vi "Host_HealthCheck_update.vi"(0 "reference in":refnum<vi>, 1 "input cluster":T1={"cRIO Data"={"Time (ms)"=0.0, "24V Battery (V)"=0.0, "LowV Current (A)"=0.0, "Fiducial Sensor (V)"=0.0, "PV Pressure (psig)"=0.0, "Flow Sensor (V)"=0.0, "Temp Fairing (F)"=0.0, "Temp Reservoir (F)"=0.0, "HallEffect Right (in)"=0.0, "HallEffect Left (in)"=0.0, "PT Tank (psig)"=0.0, "PT Clamp Right (psig)"=0.0, "PT Clamp Left (psig)"=0.0, "PT Brake (psig)"=0.0, "PT Cooling (psig)"=0.0, "Displacement (ft)"=0.0, "Velocity (ft/s)"=0.0}, "IMU Data"={"x acceleration (g)"=0.0, "Pressure (psia)"=0.0, "Temperature (F)"=0.0}, "BMS Data"={"Max Cell Voltage (V)"=0.0, "Max Cell ID"=0.0, "Min Cell Voltage (V)"=0.0, "Min Cell ID"=0.0, "State of Charge (%)"=0.0, "Average Voltage (V)"=0.0, "Voltage Delta (V)"=0.0, "Pack Current (A)"=0.0, "Pack Voltage (V)"=0.0, "Max Resistance (Ohm)"=0.0, "Min Resistance (Ohm)"=0.0, "Average Resistance (Ohm)"=0.0, "Delta Resistance (Ohm)"=0.0, "Highest Temperature(F)"=0.0, "BmsStatus"={"isFault"=FALSE, "isolationMonitoring"=FALSE}}, "Motor Data"={"Velo (RPM)"=0.0, "MotorTemp(F)"=0.0, "CtrlTemp(F)"=0.0, "DcLinkVolt(V)"=0.0, "ErrorCode"=0.0, "motorStatus"={"isReady"=FALSE, "isOn"=FALSE, "isOperEn"=FALSE, "isFault"=FALSE, "isVoltEn"=FALSE, "targetReached"=FALSE, "isWarning"=FALSE}, "isAlive"=FALSE, "motorControllerState"=1}} {"Motor Data"."motorControllerState" items=["unknown"=1, "boot-up"=0, "stopped"=4, "operational"=5, "pre-operational"=127, "connection lost"=128]}) -> ()   [LabVIEW 2017]
doc: "Updates Health Check Display\nIN: Table, Sensor Data\nOUT: Updated Table"
uses:
  Master/DAQ/Master_DataControl.ctl
  Master/DAQ/TypeDef_cRIOData.ctl
  Master/IMU/TypeDef_IMUData.ctl
  Master/CAN/TypeDef_BMSData.ctl
  Master/CAN/TypeDef_BMS_Status.ctl
  Master/CAN/MotorController/fixedMotorData.ctl
  Master/CAN/MotorController/MotorStatus.ctl
  <vilib>/Utility/miscctls.llb/LVRowAndColumnTypeDef.ctl
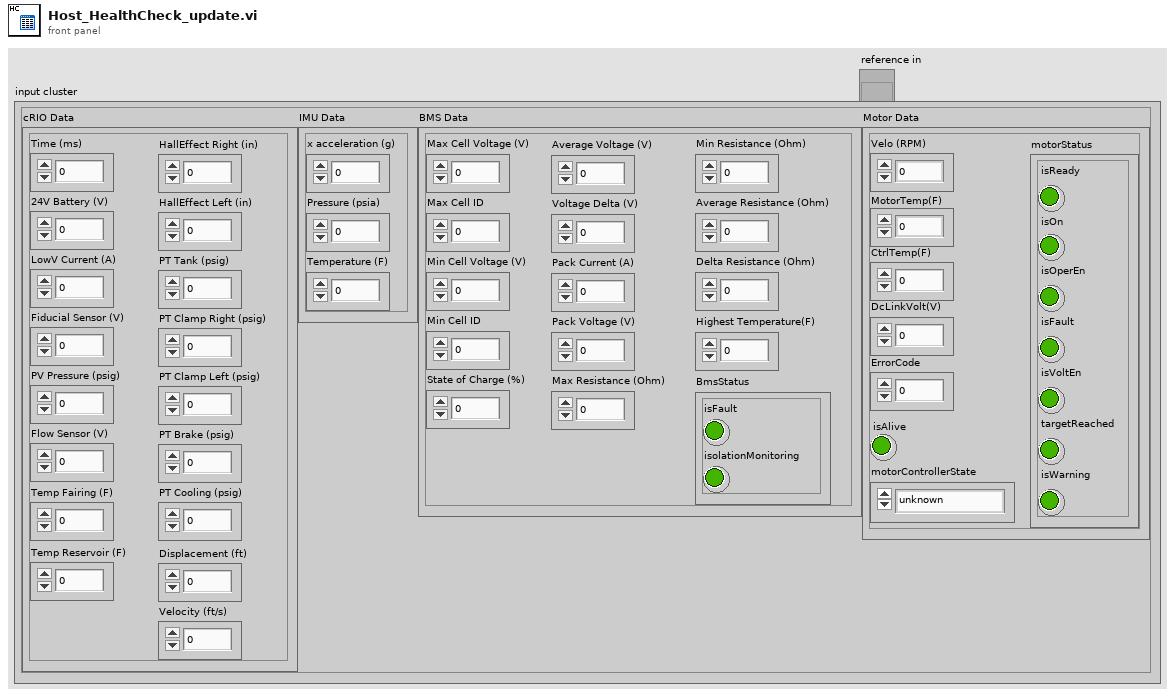
[diagram p1: front panel]
types:
  T1 = typedef "Master_DataControl.ctl" = cluster{"cRIO Data":T2, "IMU Data":T3, "BMS Data":T4, "Motor Data":T6}
  T2 = typedef "TypeDef_cRIOData.ctl" = cluster{"Time (ms)":dbl, "24V Battery (V)":dbl, "LowV Current (A)":dbl, "Fiducial Sensor (V)":dbl, "PV Pressure (psig)":dbl, "Flow Sensor (V)":dbl, "Temp Fairing (F)":dbl, "Temp Reservoir (F)":dbl, "HallEffect Right (in)":dbl, "HallEffect Left (in)":dbl, "PT Tank (psig)":dbl, "PT Clamp Right (psig)":dbl, "PT Clamp Left (psig)":dbl, "PT Brake (psig)":dbl, "PT Cooling (psig)":dbl, "Displacement (ft)":dbl, "Velocity (ft/s)":dbl}
  T3 = typedef "TypeDef_IMUData.ctl" = cluster{"x acceleration (g)":dbl, "Pressure (psia)":dbl, "Temperature (F)":dbl}
  T4 = typedef "TypeDef_BMSData.ctl" = cluster{"Max Cell Voltage (V)":dbl, "Max Cell ID":dbl, "Min Cell Voltage (V)":dbl, "Min Cell ID":dbl, "State of Charge (%)":dbl, "Average Voltage (V)":dbl, "Voltage Delta (V)":dbl, "Pack Current (A)":dbl, "Pack Voltage (V)":dbl, "Max Resistance (Ohm)":dbl, "Min Resistance (Ohm)":dbl, "Average Resistance (Ohm)":dbl, "Delta Resistance (Ohm)":dbl, "Highest Temperature(F)":dbl, "BmsStatus":T5}
  T5 = typedef "TypeDef_BMS_Status.ctl" = cluster{"isFault":bool, "isolationMonitoring":bool}
  T6 = typedef "fixedMotorData.ctl" = cluster{"Velo (RPM)":dbl, "MotorTemp(F)":dbl, "CtrlTemp(F)":dbl, "DcLinkVolt(V)":dbl, "ErrorCode":dbl, "motorStatus":T7, "isAlive":bool, "motorControllerState":u16}
  T7 = typedef "MotorStatus.ctl" = cluster{"isReady":bool, "isOn":bool, "isOperEn":bool, "isFault":bool, "isVoltEn":bool, "targetReached":bool, "isWarning":bool}
  T8 = typedef "LVRowAndColumnTypeDef.ctl" = cluster{"Row":i32, "Column":i32}
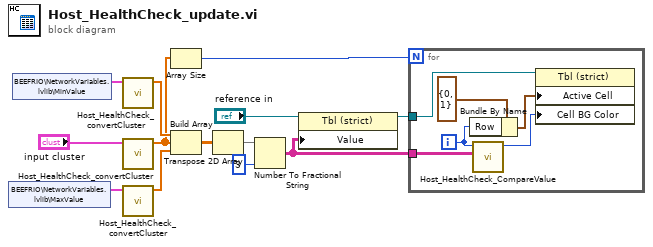
[diagram p0: block diagram]
diagram:
  n1 = shared-variable "BEEFRIO\\NetworkVariables.lvlib\\MaxValue"() -> (w2:T1)  [unwired: 1 in, 1 out]
  n2 = shared-variable "BEEFRIO\\NetworkVariables.lvlib\\MinValue"() -> (w1:T1)  [unwired: 1 in, 1 out]
  n3 = call "Host_HealthCheck_convertCluster.vi"("Data"=w1) -> ("Array"=w8:dbl[])  [unwired: 10 in]
  n4 = call "Host_HealthCheck_convertCluster.vi"("Data"="input cluster") -> ("Array"=w6:dbl[])  [unwired: 10 in]
  n5 = call "Host_HealthCheck_convertCluster.vi"("Data"=w2) -> ("Array"=w7:dbl[])  [unwired: 10 in]
  n6 = Array Size(array=w6) -> (size(s)=w13:i32)
  n7 = Build Array(w8, w6, w7) -> (w9:dbl[][])
  n8 = Transpose 2D Array(2D array=w9) -> (transposed array=w10:dbl[][])
  n9 = Number To Fractional String(number=w10, precision (6)=i16 3) -> (F-format string=w5:string[][])  [unwired: 2 in]
  n10 = property on="Property Node" class="Tbl (strict)"(reference="reference in", "Value"=w5) -> (reference out=w4:refnum<vi>)  [unwired: 1 in, 1 out]
  n11 = for {
    N: w13 -> [_]
    tunnel: w5 -> [w16]
    tunnel: w4 -> [w14]
    i -> [w15]
    n12 = Bundle By Name(cluster=T8 {"Row"=0, "Column"=1} ("Active Cell:Active Cell"), "Row"=w15) -> (w18:T8)
    n13 = call "Host_HealthCheck_CompareValue.vi"("Table in"=w16, "Index"=w15) -> ("r/g"=w19:u32)  [unwired: 9 in]
    n14 = property on="Property Node" class="Tbl (strict)"(reference=w14, "Active Cell"=w18, "Cell BG Color"=w19) -> ()  [unwired: 1 in, 2 out]
  }
